vi "pressure.vi"(8 "error in (no error)":errorcluster, 11 "VISA resource name":refnum<visa-resource-name>) -> (0 "error out":errorcluster, 2 "Pressure":dbl, 3 "VISA resource name out":refnum<visa-resource-name>)   [LabVIEW 2023]
uses:
  <vilib>/Utility/error.llb/Trim Whitespace One-Sided.vi
panel:
  out "Waveform Chart":dbl(graph)
  out "Meas result":string
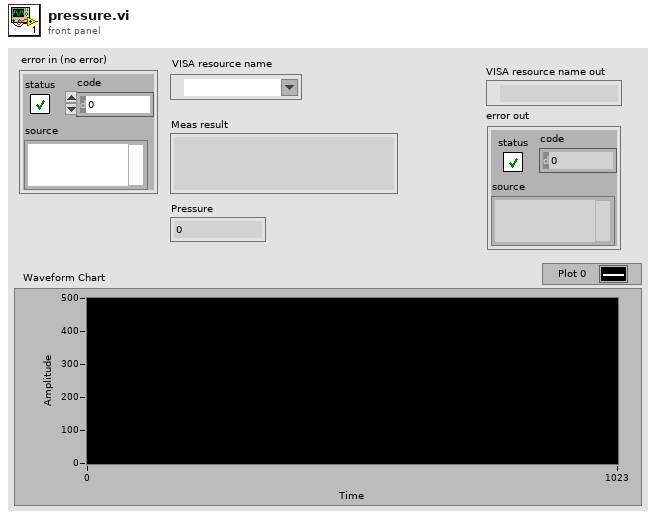
[diagram p1: front panel]
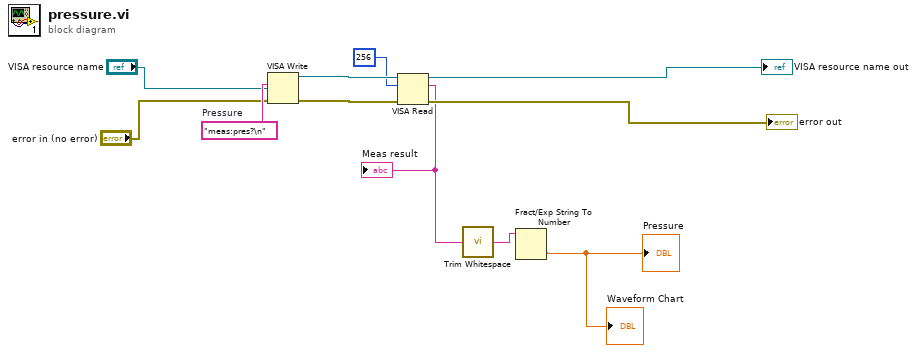
[diagram p0: block diagram]
diagram:
  w8 = "meas:pres?\n"  # Pressure
  n1 = VISA Write(VISA resource name="VISA resource name", write buffer=w8, error in (no error)="error in (no error)") -> (VISA resource name out=w11:refnum<visa-resource-name>, error out=w10:errorcluster)  [unwired: 1 out]
  n2 = VISA Read(VISA resource name=w11, byte count=u32 256, error in (no error)=w10) -> (VISA resource name out=→"VISA resource name out":refnum<visa-resource-name>, read buffer=w2:string, error out=→"error out":errorcluster)  [unwired: 1 out]
  "Meas result" <- w2
  n3 = call <vilib>:"Trim Whitespace.vi"("string"=w2) -> ("trimmed string"=w3:string)  [unwired: 1 in]
  n4 = Fract/Exp String To Number(string=w3) -> (number=→"Pressure" →"Waveform Chart":dbl)  [unwired: 3 in, 1 out]
